vi "Send FFT Data To Network Client.vi"(8 "error in (no error)":errorcluster) -> (0 "error out":errorcluster)   [LabVIEW 2016]
doc: "Sends the processed FFT data to a connected client for display."
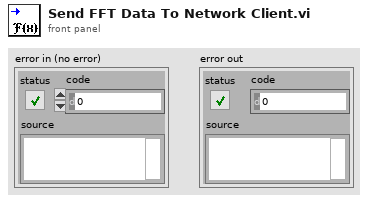
[diagram p1: front panel]
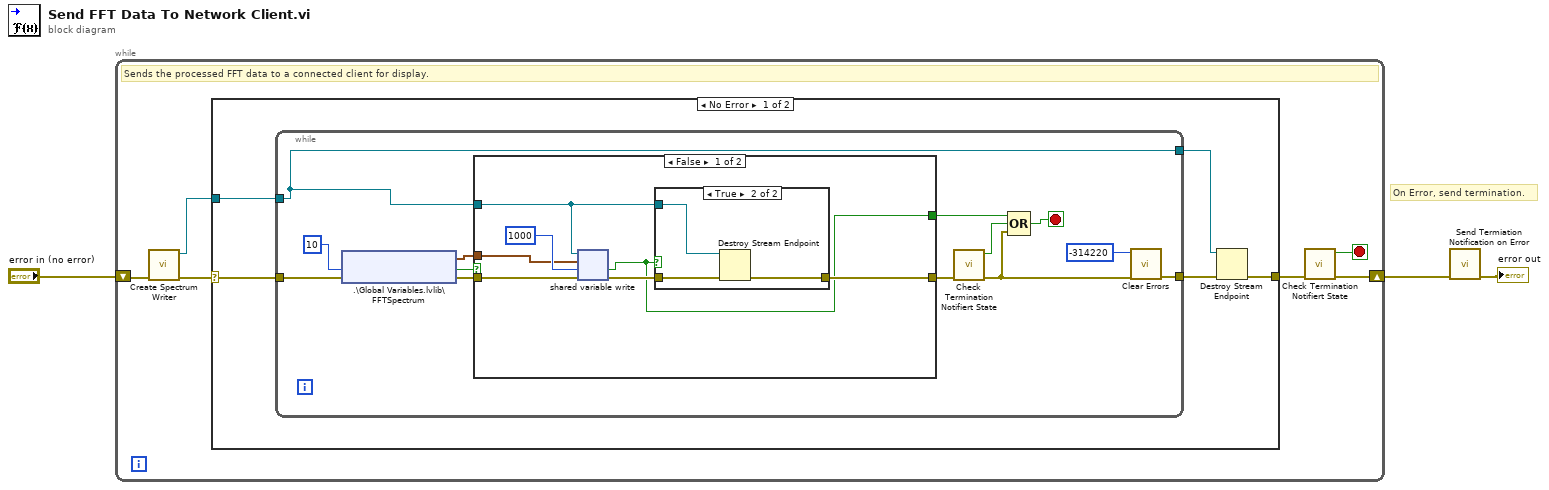
[diagram p0: block diagram]
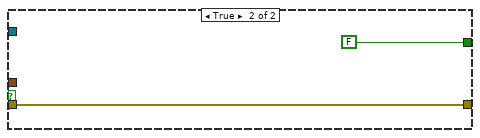
[diagram p3: hidden frame]
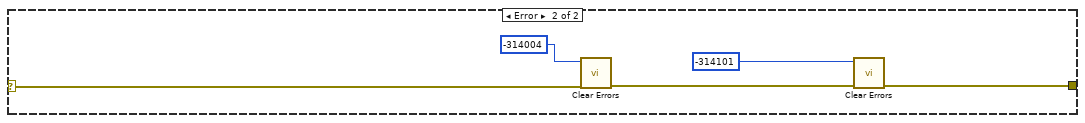
[diagram p4: hidden frame]
diagram:
  # "On Error, send termination."
  n1 = while {
    shift-right: [w4] -> w2
    shift-left: "error in (no error)" -> [w9]
    stop <- w7 stop-if-true
    # "Sends the processed FFT data to a connected client for display."
    n2 = call "Create Spectrum Writer.vi"("error in (no error)"=w9) -> ("error out"=w8:errorcluster, "Writer"=w6:refnum<k21>)  [unwired: 9 in]
    n3 = case shown="No Error" w8 {
      selector: w8 -> [w14 w41]
      tunnel: [w11 w45] -> w5
      tunnel: w6 -> [w13 _]
      frame No Error {
        n4 = while {
          tunnel: w14 -> [w19]
          tunnel: [w24] -> w12
          tunnel: w13 -> [w21]
          tunnel: [w21] -> w10
          stop <- w25 stop-if-true
          n5 = shared-variable ".\\Global Variables.lvlib\\FFTSpectrum"(error in=w19, 10 ("ms timeout (0)")) -> (w15:waveform(dbl), error out=w18:errorcluster, w16:bool)
          n6 = case shown="False" w16 {
            tunnel: w18 -> [w34 w39]
            tunnel: w15 -> [w29 _]
            tunnel: [w32 w39] -> w27
            tunnel: w21 -> [w28 _]
            tunnel: [w31 FALSE] -> w20
            frame False {
              n7 = shared-variable-write(w28, w34, w29, 1000 ("timeout ms (-1)")) -> (w33:errorcluster, w31:bool)  [unwired: 1 out]
              n8 = case shown="True" w31 {
                tunnel: w33 -> [w35 w38]
                tunnel: w28 -> [_ w37]
                tunnel: [w35 w36] -> w32
                frame False {
                }
                frame True {
                  n9 = Destroy Stream Endpoint(8:w38, 11:w37) -> (0:w36:errorcluster)
                }
              }
            }
            frame True {
            }
          }
          n10 = call "Check Termination Notifiert State.vi"("error in (no error)"=w27) -> ("error out"=w22:errorcluster, "Termination Notifier State"=w26:bool)  [unwired: 9 in]
          n11 = Compound Arithmetic op=OR(w20, w26, w22) -> (w25:bool)
          n12 = call <vilib>:"Clear Errors.vi"("error in (no error)"=w22, "specific error code to clear (0: all)"=-314220) -> ("error out"=w24:errorcluster)  [unwired: 4 in, 1 out]
        }
        n13 = Destroy Stream Endpoint(8:w12, 11:w10) -> (0:w11:errorcluster)
      }
      frame Error {
        n14 = call <vilib>:"Clear Errors.vi"("error in (no error)"=w41, "specific error code to clear (0: all)"=-314004 ("y")) -> ("error out"=w43:errorcluster)  [unwired: 4 in, 1 out]
        n15 = call <vilib>:"Clear Errors.vi"("error in (no error)"=w43, "specific error code to clear (0: all)"=-314101) -> ("error out"=w45:errorcluster)  [unwired: 4 in, 1 out]
      }
    }
    n16 = call "Check Termination Notifiert State.vi"("error in (no error)"=w5) -> ("error out"=w4:errorcluster, "Termination Notifier State"=w7:bool)  [unwired: 9 in]
  }
  n17 = call "Send Termiation Notification on Error.vi"("error in (no error)"=w2) -> ("error out"=→"error out":errorcluster)  [unwired: 10 in]
